vi "Write Value (variant).vi"(8 "error in (no error)":errorcluster, 10 "Variant":variant, 11 "Double D Element in":refnum<class "Double D Element.lvclass">) -> (0 "error out":errorcluster, 3 "Double D Element out":refnum<class "Double D Element.lvclass">)   [LabVIEW 2018, in "D Datagrid Library.lvlib" / "Double D Element.lvclass"]
uses:
  Double D Element.lvclass
  Double D Element.lvclass/Double D Element.ctl
  Write Value.vi
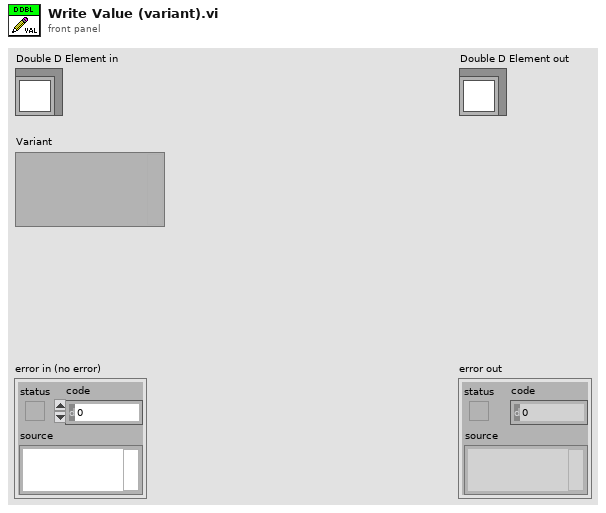
[diagram p1: front panel]
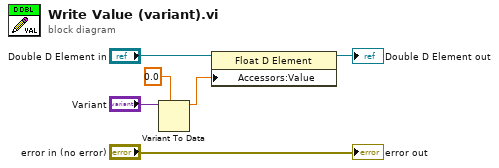
[diagram p0: block diagram]
diagram:
  n1 = Variant To Data(type=0.0 ("Value"), Variant="Variant") -> (data=w1:dbl)  [unwired: 1 in, 1 out]
  n2 = property class="Float D Element"(reference="Double D Element in", "Accessors:Value"=w1) -> (reference out=→"Double D Element out":refnum<class "Double D Element.lvclass">)  [unwired: 1 in, 1 out]
  "error out" <- "error in (no error)"
